vi "Exemple_Preprocessing_maxabs_scale.vi"() -> ()   [LabVIEW 2020]
panel:
  out "Data":T1
  out "error out":errorcluster
  in  "X":string[][](array[string])=[["1", "-1", "2"], ["2", "0", "0"], ["0", "1", "-1"]]
  in  "error in":errorcluster caption="entrée d'erreur"
  in  "maxabs_scale":cluster{"axis":i32, "copy":bool}={"axis"=0, "copy"=TRUE}
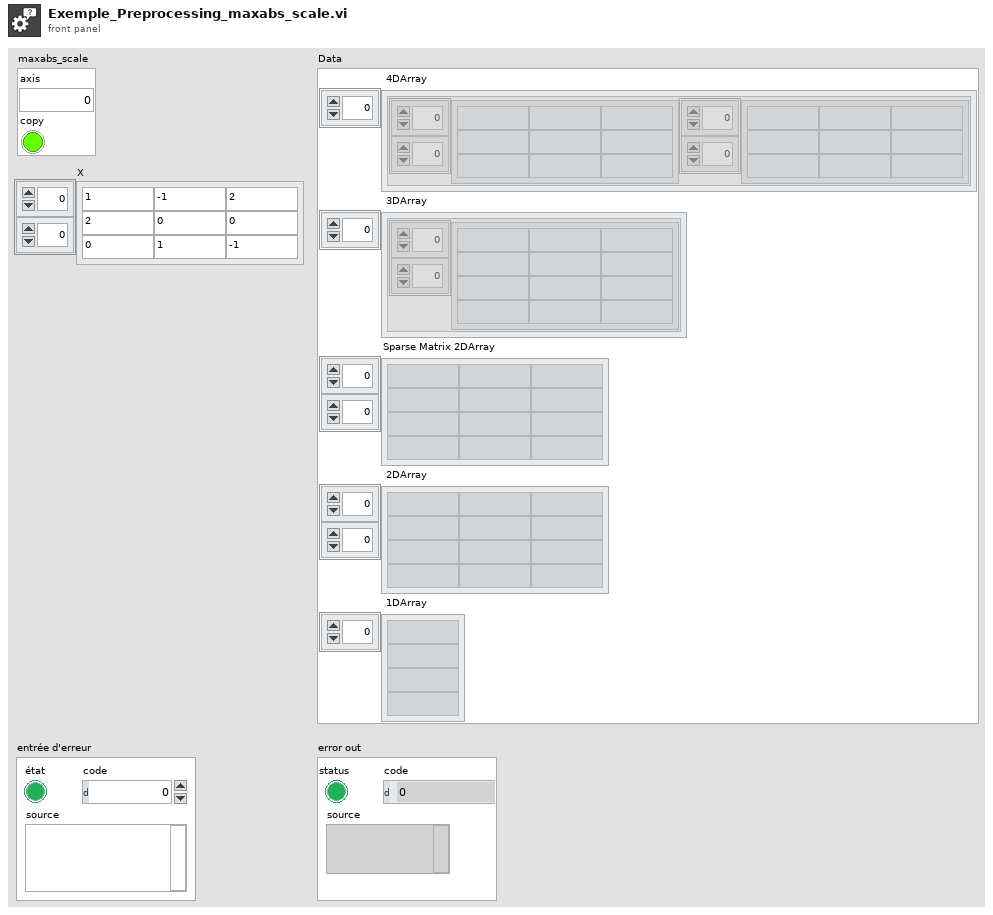
[diagram p1: front panel]
types:
  T1 = cluster{" 4DArray":cluster{"1":string[][], "2":string[][]}[], " 3DArray":cluster{"Tableau":string[][]}[], "Sparse Matrix 2DArray":string[][], " 2DArray":string[][], " 1DArray":string[]}
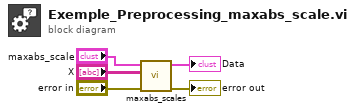
[diagram p0: block diagram]
diagram:
  n1 = call "maxabs_scales.vi"("error in"="error in", "X"="X", "maxabs_scale"="maxabs_scale") -> ("error out"=→"error out":errorcluster, "Data"=→"Data":T1)  [unwired: 7 in]
